vi "Create New Class.vi"(8 "Error In":errorcluster, 9 "Class Path":path, 10 "Class Name":string, 11 "Base Class":refnum<vi>) -> (0 "Error Out":errorcluster, 1 "Class Path Dup":path, 2 "New Class":refnum<vi>)   [LabVIEW 2013]
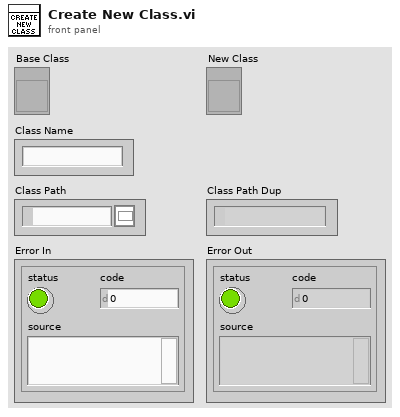
[diagram p1: front panel]
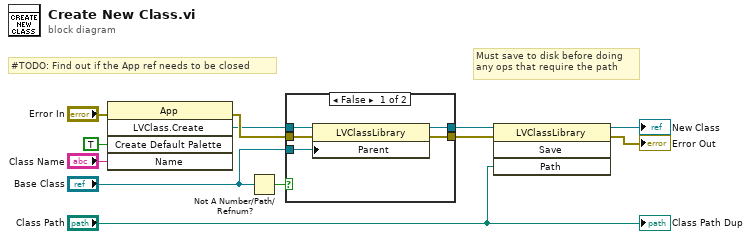
[diagram p0: block diagram]
diagram:
  # "Must save to disk before doing\nany ops that require the path"
  # "#TODO: Find out if the App ref needs to be closed"
  n1 = invoke class="App" method="LVClass.Create"(error in="Error In", "Create Default Palette"=TRUE ("Create:Default Palette"), "Name"="Class Name") -> (error out=w12:errorcluster, "LVClass.Create"=w11:refnum<vi>)  [unwired: 2 in, 3 out]
  n2 = Not A Number/Path/Refnum?(number/path/refnum="Base Class") -> (NaN/Path/Refnum?=w10:bool)
  n3 = case shown="False" w10 {
    tunnel: w11 -> [w17 w18]
    tunnel: "Base Class" -> [w16 _]
    tunnel: w12 -> [w15 w19]
    tunnel: [w14 w18] -> w5
    tunnel: [w13 w19] -> w3
    frame False {
      n4 = property class="LVClassLibrary"(reference=w17, error in=w15, "Parent"=w16) -> (reference out=w14:refnum<vi>, error out=w13:errorcluster)
    }
    frame True {
    }
  }
  n5 = invoke class="LVClassLibrary" method="Save"(reference=w5, error in=w3, "Path"="Class Path") -> (reference out=→"New Class":refnum<vi>, error out=→"Error Out":errorcluster)  [unwired: 1 in, 2 out]
  "Class Path Dup" <- "Class Path"
